vi "Scan Engine Update Slot Subpanel.vi"(7 "SubPanel Event":refnum<user-event>, 8 "error in (no error)":errorcluster, 9 "SubPanel Ref":refnum<vi>, 10 "RSI Module in":refnum<class "RSI Module.lvclass">=refnum, 11 "Node Ptr In":T1 format="%.0x") -> (0 "error out":errorcluster, 2 "RSI Module out":refnum<class "RSI Module.lvclass">, 3 "Node Ptr Out":T1 format="%.0x")   [LabVIEW 2016, in "Scan Engine Custom Device.lvlib"]
uses:
  Scan Engine Custom Device.lvlib
  Modules.lvlibp/RSI Module/RSI Module.lvclass
  <vilib>/Utility/miscctls.llb/LVRectTypeDef.ctl
  Globals/SubPanel Controls.vi
  <vilib>/NI Veristand/Custom Device API/Custom Device Item Ref.ctl
  <vilib>/NI Veristand/Custom Device API/Custom Device API.lvlib
  Modules.lvlibp/RSI Module/SubPanel Command.ctl
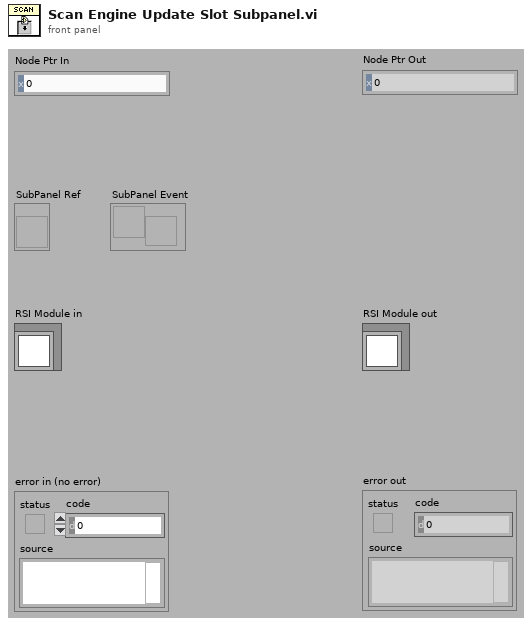
[diagram p1: front panel]
types:
  T1 = typedef "Custom Device API.lvlib/Custom Device Item Ref.ctl" = u64
  T2 = typedef "LVRectTypeDef.ctl" = cluster{"Left":i16, "Top":i16, "Right":i16, "Bottom":i16}
  T3 = typedef "LVBoundsTypeDef.ctl" = cluster{"Width":u32, "Height":u32}
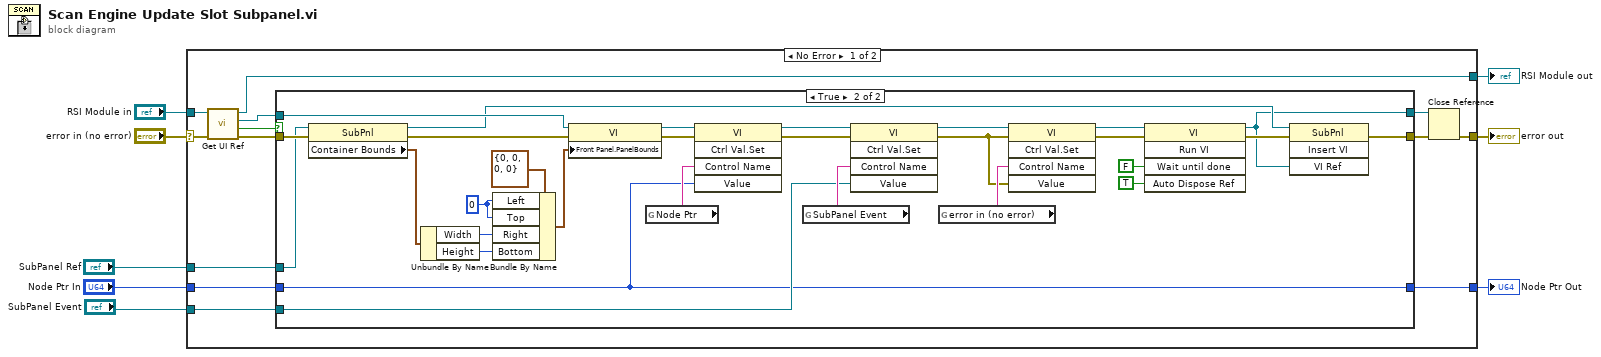
[diagram p0: block diagram]
diagram:
  n1 = case shown="No Error" "error in (no error)" {
    selector: "error in (no error)" -> [w11 w56]
    tunnel: "SubPanel Ref" -> [w21 _]
    tunnel: [w17 w56] -> w7
    tunnel: "Node Ptr In" -> [w16 w55]
    tunnel: "SubPanel Event" -> [w14 _]
    tunnel: "RSI Module in" -> [w13 w54]
    tunnel: [w12 w54] -> w4
    tunnel: [w9 w55] -> w2
    frame No Error {
      n2 = call-dynamic "Get UI Ref.vi"("error in (no error)"=w11, "RSI Module in"=w13) -> ("error out"=w15:errorcluster, "Show SubPanel?"=w10:bool, "VI Refnum"=w20:refnum<vi>, "RSI Module out"=w12:refnum<class "RSI Module.lvclass">)  [unwired: 6 in]
      n3 = case shown="True" w10 {
        tunnel: w21 -> [_ w31]
        tunnel: w20 -> [w23 w48]
        tunnel: [w23 w25] -> w19
        tunnel: [w24 w26] -> w18
        tunnel: w16 -> [w22 w32]
        tunnel: w15 -> [w24 w36]
        tunnel: w14 -> [_ w33]
        tunnel: [w22 w32] -> w9
        frame False {
        }
        frame True {
          w51 = i16 0 ("Left")
          n4 = property class="SubPnl"(reference=w31, error in=w36) -> (reference out=w28:refnum<vi>, error out=w35:errorcluster, "Container Bounds"=w49:T3)
          n5 = Unbundle By Name(w49) -> ("Width"=w52:u32, "Height"=w53:u32)
          n6 = Bundle By Name(cluster=T2 {"Left"=0, "Top"=0, "Right"=0, "Bottom"=0} ("Front Panel Window:Panel Bounds"), "Left"=w51, "Top"=w51, "Right"=w52, "Bottom"=w53) -> (w47:T2)
          n7 = property class="VI"(reference=w48, error in=w35, "Front Panel.PanelBounds"=w47) -> (reference out=w46:refnum<vi>, error out=w45:errorcluster)
          n8 = global read "SubPanel Controls.vi" "Node Ptr"() -> (w37:string)
          n9 = invoke class="VI" method="Ctrl Val.Set"(reference=w46, error in=w45, "Control Name"=w37, "Value"=w32) -> (reference out=w44:refnum<vi>, error out=w43:errorcluster)  [unwired: 1 in, 3 out]
          n10 = global read "SubPanel Controls.vi" "SubPanel Event"() -> (w34:string)
          n11 = invoke class="VI" method="Ctrl Val.Set"(reference=w44, error in=w43, "Control Name"=w34, "Value"=w33) -> (reference out=w30:refnum<vi>, error out=w29:errorcluster)  [unwired: 1 in, 3 out]
          n12 = global read "SubPanel Controls.vi" "error in (no error)"() -> (w38:string)
          n13 = invoke class="VI" method="Ctrl Val.Set"(reference=w30, error in=w29, "Control Name"=w38, "Value"=w29) -> (reference out=w42:refnum<vi>, error out=w41:errorcluster)  [unwired: 1 in, 3 out]
          n14 = invoke class="VI" method="Run VI"(reference=w42, error in=w41, "Wait until done"=FALSE ("Wait Until Done"), "Auto Dispose Ref"=TRUE ("Auto Dispose Reference")) -> (reference out=w25:refnum<vi>, error out=w27:errorcluster)  [unwired: 1 in, 3 out]
          n15 = invoke class="SubPnl" method="Insert VI"(reference=w28, error in=w27, "VI Ref"=w25) -> (error out=w26:errorcluster)  [unwired: 1 in, 3 out]
        }
      }
      n16 = Close Reference(reference=w19, error in (no error)=w18) -> (error out=w17:errorcluster)
    }
    frame Error {
    }
  }
  "error out" <- w7
  "Node Ptr Out" <- w2
  "RSI Module out" <- w4
